vi "Detector Make FITS Templates.vi"(8 "error in (no error)":errorcluster, 11 "RIMAS Detector in":refnum<class "Obsolete Detector.lvclass">) -> (0 "error out":errorcluster, 3 "RIMAS Detector out":refnum<class "Obsolete Detector.lvclass">)   [LabVIEW 2022 SP3, in "Obsolete Detector.lvclass"]
uses:
  Obsolete Detector.lvclass
  Detector Class.lvclass
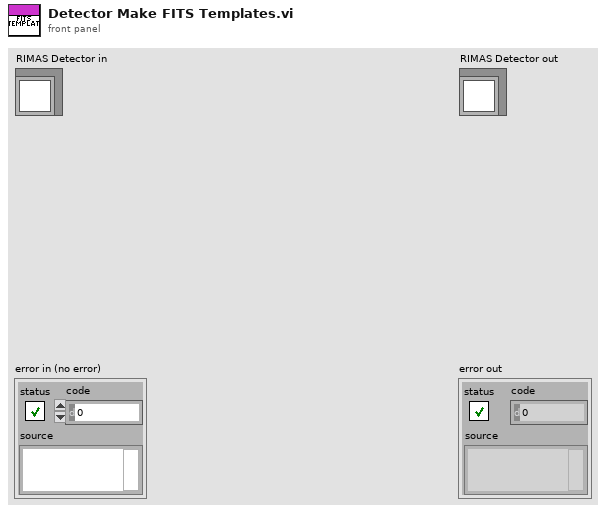
[diagram p1: front panel]
types:
  T1 = typedef "RIMAS Detector Config.ctl" = cluster{"Detector":u16, "Offsets":u16[][], "Detector Computer":T2, "FITS hdr template0":path, "FITS hdr template1":path, "FITS Data File Path":path, "FITS Detector Settings":T3, "Sim Folder":path, "Integration Mode":T4, "Integration Time":dbl, "Frame Int Time":dbl}
  T2 = typedef "RIMAS Detector Server Config.ctl" = cluster{"Machine":string, "Password":string, "FITS File Path":string, "Port":u16, "Header Path":string, "Name":string}
  T3 = typedef "RIMAS Observation Config.ctl" = cluster{"Exp Time Short":dbl, "# of Frames":dbl, "Exp Time Long":dbl, "# of Groups":dbl, "Object Name":string, "Object":string, "Obs Type":string, "Image Type":string, "Observer":string, "Observer Affiliation":string}
  T4 = typedef "Detector enum Detector Integration Mode.ctl" = enum16{"SSR", "CDS", "MEAN", "MEDIAN", "MODE", "MIIN", "MAX"}
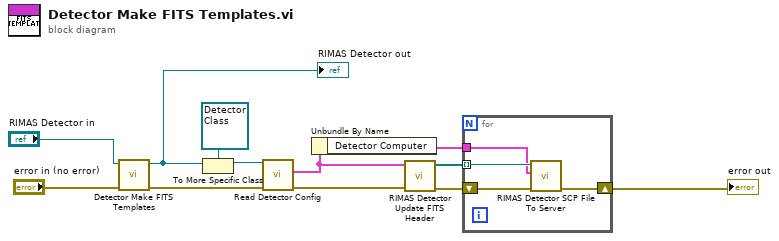
[diagram p0: block diagram]
diagram:
  n1 = call-parent "Detector Make FITS Templates.vi"("error in (no error)"="error in (no error)", "Detector Class in"="RIMAS Detector in") -> ("error out"=w8:errorcluster, "Detector Class out"=w1:refnum<class "Obsolete Detector.lvclass">)  [unwired: 8 in]
  "RIMAS Detector out" <- w1
  n2 = To More Specific Class(target class=refnum<class "Detector Class.lvclass"> refnum ("Detector Class.lvclass"), reference=w1) -> (specific class reference=w9:refnum<class "Detector Class.lvclass">)  [unwired: 1 in, 1 out]
  n3 = call-dynamic "Read Detector Config.vi"("error in (no error)"=w8, "Detector Class in"=w9) -> ("error out"=w4:errorcluster, "Detector Config"=w5:T1)  [unwired: 7 in, 1 out]
  n4 = Unbundle By Name(w5) -> ("Detector Computer"=w3:T2)
  n5 = call "RIMAS Detector Update FITS Header.vi"("Error In"=w4, "Detector Config"=w5) -> ("Error Out"=w6:errorcluster, "Files"=w7:path[])  [unwired: 8 in]
  n6 = for {
    tunnel: w7 -> [w16] mode=indexing
    tunnel: w3 -> [w15]
    shift-right: [w13] -> w2
    shift-left: w6 -> [w14]
    n7 = call "RIMAS Detector SCP File To Server.vi"("Error In"=w14, "Detector Computer"=w15, "Local File Path"=w16) -> ("Error Out"=w13:errorcluster)  [unwired: 7 in, 1 out]
  }
  "error out" <- w2
